vi "Get All Columns.vi"(11 "error in (no error)":errorcluster) -> (4 "All Columns out":cluster{string, i32}[](array[cluster]), 15 "error out":errorcluster)   [LabVIEW 2023, in "RFCalAndFixtureCharact.Common.lvlib"]
uses:
  RFCalAndFixtureCharact.Common.lvlib
  Type Definitions/Dictionary Operation.ctl
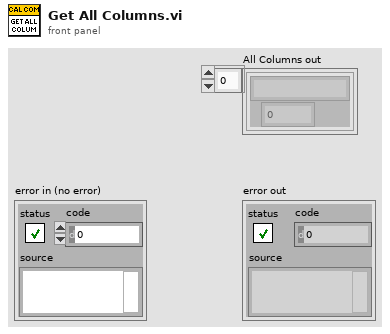
[diagram p1: front panel]
types:
  T1 = typedef "RFCalAndFixtureCharact.Common.lvlib/Dictionary Operation.ctl" = enum16{"Read", "Insert", "Remove", "Clear", "Get All", "Update"}
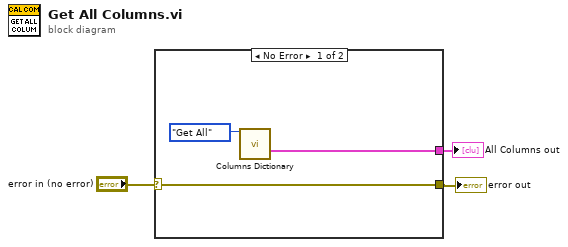
[diagram p0: block diagram]
diagram:
  n1 = case shown="No Error" "error in (no error)" {
    selector: "error in (no error)" -> [w5 w7]
    tunnel: [w5 w7] -> w2
    tunnel: [w4 _] -> w1
    frame No Error {
      n2 = call "Columns Dictionary.vi"("Action"=Dictionary_Operation."Get All") -> ("Columns"=w4:cluster{string, i32}[])  [unwired: 12 in, 2 out]
    }
    frame Error {
    }
  }
  "error out" <- w2
  "All Columns out" <- w1
